vi "New.vi"(8 "error in (no error)":errorcluster, 9 "ErrorOrSuccess JSON":refnum<class "ErrorOrSuccess JSON.lvclass">, 10 "SubscriptionDetails JSON":refnum<class "SubscriptionDetails JSON.lvclass">, 11 "Topic":string) -> (0 "error out":errorcluster, 3 "SubscribeResult JSON out":refnum<class "SubscribeResult JSON.lvclass">)   [LabVIEW 2020, in "wamplv.lvlib" / "SubscribeResult JSON.lvclass"]
uses:
  SubscribeResult JSON.lvclass
  SubscribeResult JSON.lvclass/SubscribeResult JSON.ctl
  Private/Message loop classes/ErrorOrSuccess JSON/ErrorOrSuccess JSON.lvclass
  Private/Message loop classes/Subscription details/SubscriptionDetails JSON/SubscriptionDetails JSON.lvclass
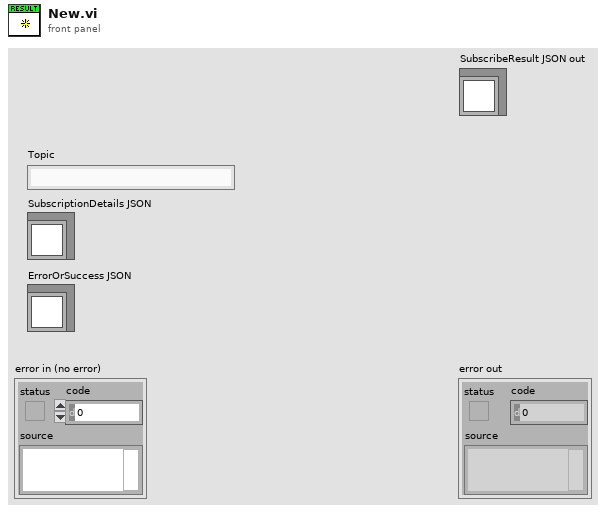
[diagram p1: front panel]
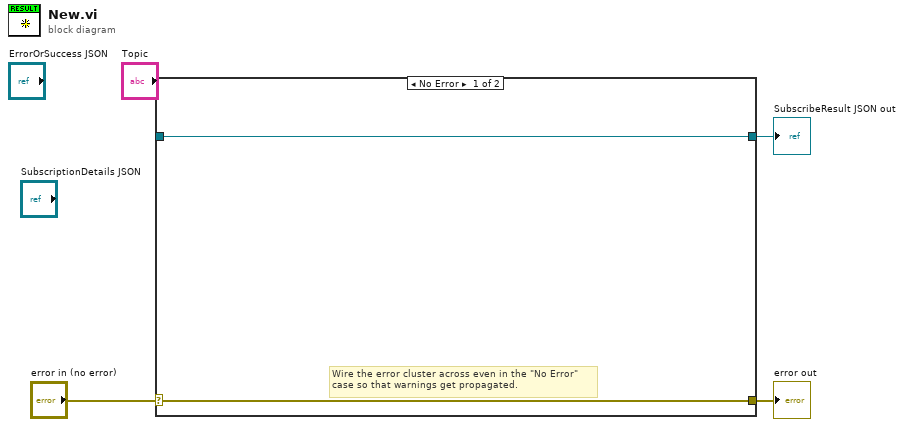
[diagram p0: block diagram]
diagram:
  n1 = case shown="No Error" "error in (no error)" {
    selector: "error in (no error)" -> [w5 w8]
    tunnel: [w5 w8] -> w3
    tunnel: [w6 w7] -> w1
    tunnel: [w6 w7] -> w2
    frame No Error {
      # "Wire the error cluster across even in the \"No Error\"\ncase so that warnings get propagated."
    }
    frame Error {
    }
  }
  "error out" <- w3
  "SubscribeResult JSON out" <- w1
